vi "Main_FPGA 5.vi"() -> ()   [LabVIEW 2015]
uses:
  <vilib>/rvi/Emulation/niFpgaGetClockAttributes.vi
  <vilib>/rvi/Emulation/niFpgaSctlEmulationGetInTimedLoop.vi
  <vilib>/rvi/Emulation/niFpgaEmulationReportErrorSimple.vi
  <vilib>/rvi/Emulation/niFpgaProcessEmulError.vi
  <vilib>/rvi/eio/common/nirviEmuTemplateMethod_errors.vi
  <vilib>/rvi/interface/RandomDataEmulation/niFpgaRandomDataHandleErrors.vi
  <vilib>/rvi/Emulation/niFpgaCriticalErrorInLSC.vi
  <vilib>/eio/EIONode/EIONode.xnode
  <vilib>/rvi/DataTransferAndStorage/Container/XNode/niFpgaContainer.xnode
  <vilib>/rvi/interface/RandomDataEmulation/nirviRandomDataFpgaReadWriteTemplate.vi
panel:
  out "Loop delay (us)":u32
  out "Chassis Temperature":sgl
  out "FPGA Error":errorcluster
  out "Finished":bool
  in  "Stop":bool
  out "Module Underflow":bool
  out "DMA FIFO Full":bool
  out "Chan Count":bool
  out "Acq Loop Ticks":u32
  out "First Read":bool
  in  "Total Avail Channels":i32=4
  in  "Data Rate [S/s]":u32=1280
  in  "Acquisition Type":enum16{"Finite Samples", "Continuous Samples"}(ring)
  in  "Samps per Chan [Finite]":i32=5120
  in  "Number of Modules":i16=1
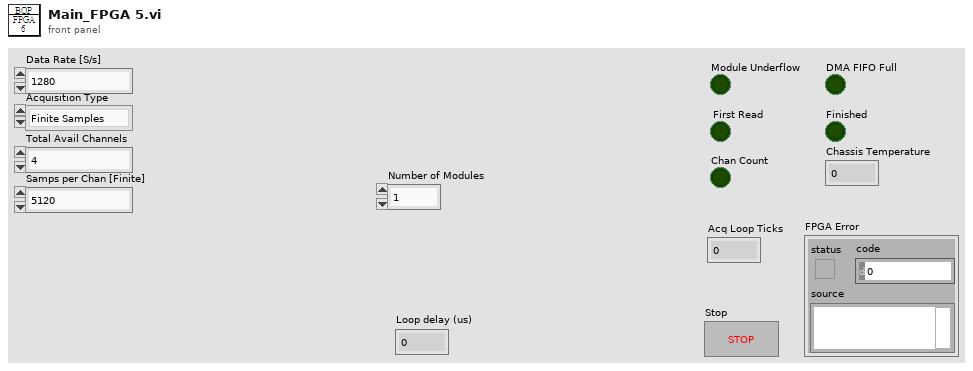
[diagram p1: front panel]
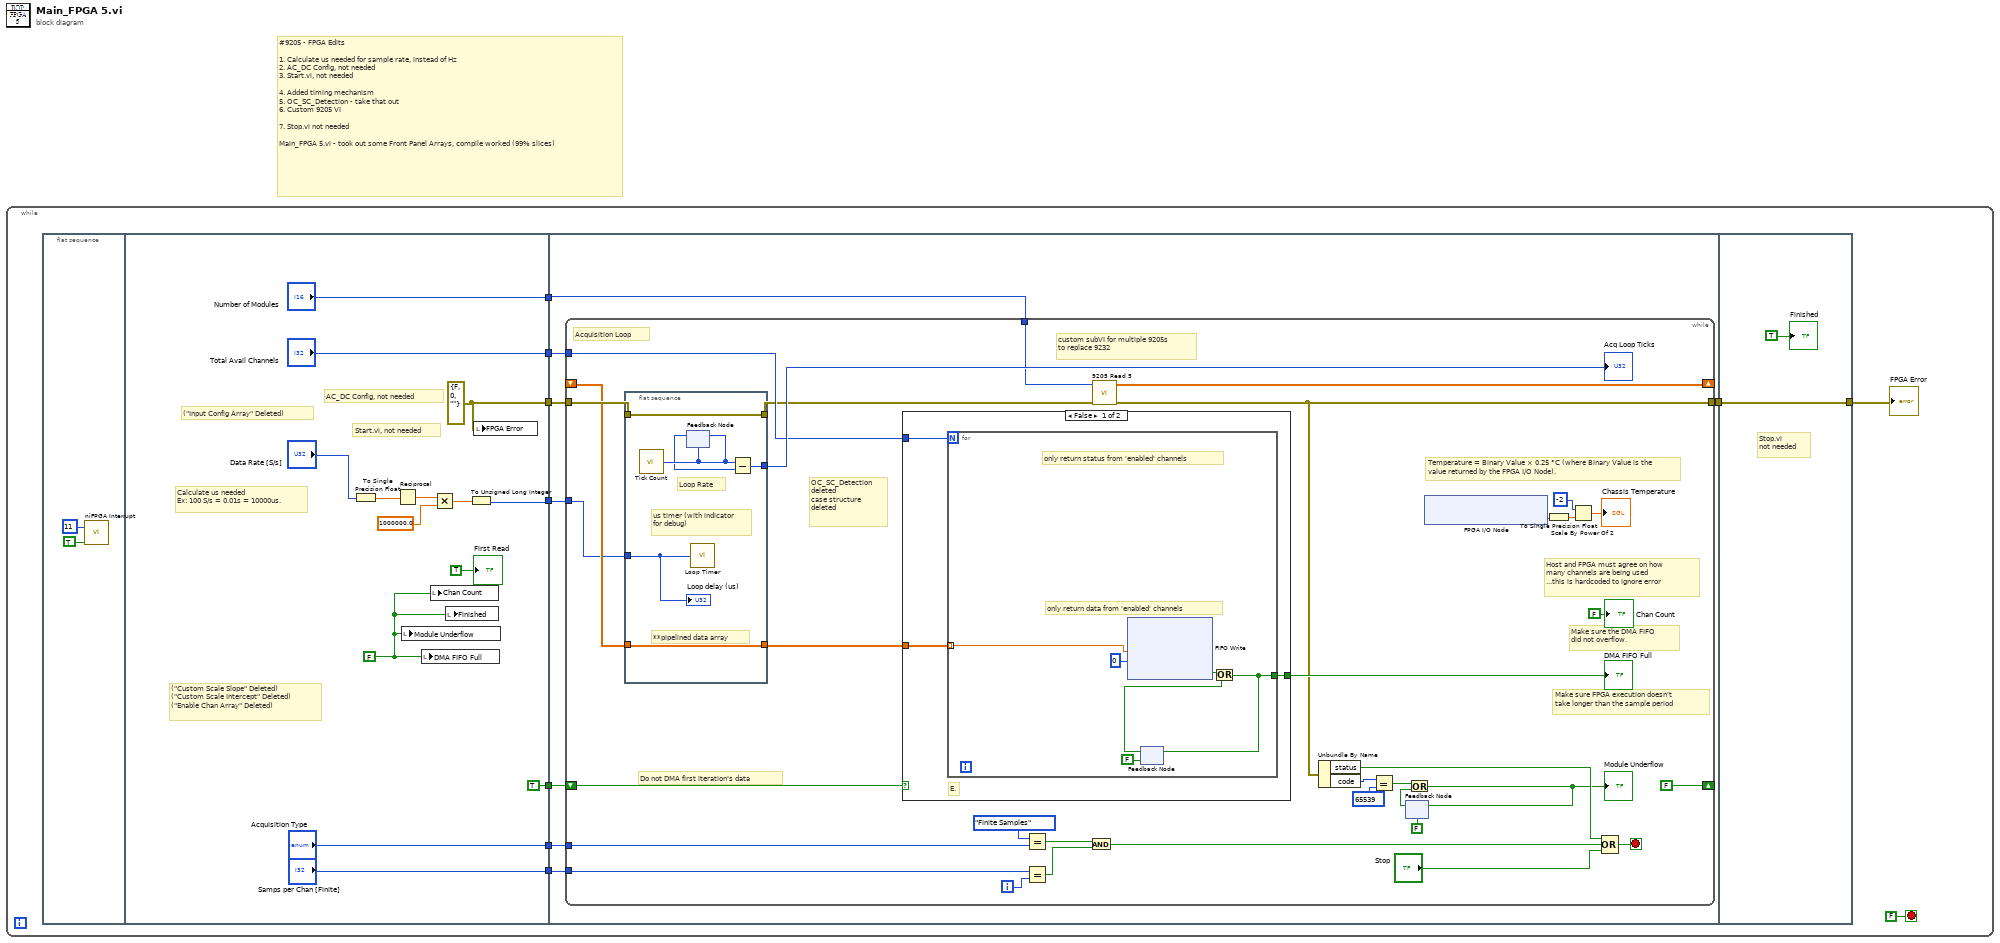
[diagram p0: block diagram]
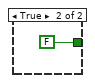
[diagram p2: hidden frame]
diagram:
  # "#9205 - FPGA Edits\n\n1. Calculate us needed for sample rate, instead of Hz\n2. AC_DC Config, not needed\n3. Start.vi, not needed\n\n4. Added timing mechanism\n5. OC_SC_Detection - take that out\n6. Custom 9205 VI\n\n7. Stop.vi not needed\n\nMain_FPGA 5.vi - took out some Front Panel Arrays, compile worked (99% slices)"
  n1 = while {
    stop <- FALSE stop-if-true
    n2 = flat-sequence {
      tunnel: [w19] -> w9
      tunnel: ["Acquisition Type"] -> w8
      tunnel: ["Samps per Chan [Finite]"] -> w7
      tunnel: ["Total Avail Channels"] -> w6
      tunnel: [TRUE ("t")] -> w5
      tunnel: ["Number of Modules"] -> w3
      tunnel: [w13] -> w1
      tunnel: w9 -> [w33]
      tunnel: w8 -> [w31]
      tunnel: w7 -> [w30]
      tunnel: w6 -> [w34]
      tunnel: w5 -> [w32]
      tunnel: [w29] -> w4
      tunnel: w3 -> [w28]
      tunnel: w1 -> [w27]
      tunnel: w4 -> [w85]
      tunnel: [w85] -> w2
      frame #0 {
        n3 = call <vilib>:"niFPGA Interrupt.vi"("Wait Until Cleared (F)"=TRUE ("Wait Until Cleared"), "IRQ Number (0)"=u8 11 ("IRQ Number")) -> ()  [unwired: 1 in]
      }
      frame #1 {
        w19 = errorcluster {"status"=FALSE, "code"=0, "source"=""} ("FPGA Error")
        w21 = FALSE ("Module Underflow")
        # "(\"Custom Scale Slope\" Deleted)\n(\"Custom Scale Intercept\" Deleted)\n(\"Enable Chan Array\" Deleted)"
        # "(\"Input Config Array\" Deleted)"
        # "Start.vi, not needed"
        # "AC_DC Config, not needed"
        # "Calculate us needed\nEx: 100 S/s = 0.01s = 10000us."
        n4 = To Single Precision Float(number="Data Rate [S/s]") -> (single precision float=w16:sgl)
        n5 = Reciprocal(x=w16) -> (1/x=w18:sgl)
        n6 = local write "Module Underflow"(w21) -> ()
        n7 = local write "DMA FIFO Full"(w21) -> ()
        n8 = local write "Chan Count"(w21) -> ()
        n9 = Multiply(x=w18, y=sgl 1000000.0) -> (x*y=w14:sgl)
        n10 = local write "Finished"(w21) -> ()
        n11 = To Unsigned Long Integer(number=w14) -> (unsigned 32bit integer=w13:u32)
        n12 = local write "FPGA Error"(w19) -> ()
        "First Read" <- TRUE ("First Read")
      }
      frame #2 {
        n13 = while {
          tunnel: w33 -> [w62]
          tunnel: [w37] -> w29
          tunnel: w31 -> [w64]
          tunnel: w30 -> [w63]
          shift-right: [w35] -> _
          shift-left: _ -> [w60]
          tunnel: w34 -> [w44]
          shift-right: [FALSE ("t")] -> _
          shift-left: w32 -> [w47]
          tunnel: w28 -> [w36]
          tunnel: w27 -> [w39]
          i -> [w58]
          stop <- w67 stop-if-true
          # "custom subVI for multiple 9205s\nto replace 9232"
          # "OC_SC_Detection\ndeleted\ncase structure\ndeleted"
          # "Temperature = Binary Value × 0.25 °C (where Binary Value is the value returned by the FPGA I/O Node)."
          # "Do not DMA first iteration's data"
          # "Acquisition Loop"
          # "Host and FPGA must agree on how \nmany channels are being used\n...this is hardcoded to ignore error"
          # "Make sure the DMA FIFO\ndid not overflow."
          # "Make sure FPGA execution doesn't\ntake longer than the sample period"
          n14 = flat-sequence {
            tunnel: [w84] -> w38
            tunnel: w62 -> [w84]
            tunnel: [w81] -> w61
            tunnel: w60 -> [w80]
            tunnel: [w80] -> w45
            tunnel: w39 -> [w79]
            frame #0 {
              # "us timer (with indicator\nfor debug)"
              # "**pipelined data array"
              # "Loop Rate"
              n15 = call "Tick Count"() -> ("Tick Count(Ticks)"=w83:u32)
              n16 = feedback-in #1(w83) -> ()
              n17 = feedback #1(w83) -> (w82:u32)
              n18 = call "Loop Timer"("Count(uSec)"=w79) -> ()  [unwired: 1 out]
              n19 = Subtract(x=w83, y=w82) -> (x-y=w81:u32)
              "Loop delay (us)" <- w79
            }
          }
          n20 = case shown="False" w47 {
            tunnel: [w71 FALSE] -> w46
            tunnel: w45 -> [w70 _]
            tunnel: w44 -> [w69 _]
            frame False {
              # "E."
              n21 = for {
                N: w69 -> [_]
                tunnel: [w76] -> w71
                tunnel: w70 -> [w75] mode=indexing
                # "only return status from 'enabled' channels"
                # "only return data from 'enabled' channels"
                n22 = xnode ("FIFO Write")("Element"=w75, "Timeout"=0) -> ("Timed Out?"=w72:bool)  [unwired: 1 in, 1 out]
                n23 = feedback #2(FALSE) -> (w77:bool)
                n24 = Or(x=w72, y=w77) -> (x .or. y?=w76:bool)
                n25 = feedback-in #2(w76) -> ()
              }
            }
            frame True {
            }
          }
          "DMA FIFO Full" <- w46
          n26 = Equal?(x=enum16{"Finite Samples", "Continuous Samples"}."Finite Samples" ("y"), y=w64) -> (x = y?=w52:bool)
          n27 = Equal?(x=w63, y=w58) -> (x = y?=w51:bool)
          n28 = And(x=w52, y=w51) -> (x .and. y?=w50:bool)
          n29 = call "9205 Read 5.vi"("error in"=w38, "Module Config Selector"=w36) -> ("error out"=w37:errorcluster, "Data Array"=w35:sgl[])  [unwired: 8 in]
          n30 = Unbundle By Name(w37) -> ("status"=w57:bool, "code"=w65:i32)
          n31 = Equal?(x=w65, y=65539) -> (x = y?=w54:bool)
          n32 = feedback #3(FALSE) -> (w56:bool)
          n33 = Or(x=w54, y=w56) -> (x .or. y?=w53:bool)
          "Module Underflow" <- w53
          n34 = feedback-in #3(w53) -> ()
          n35 = xnode "FPGA I/O Node"() -> ("Chassis Temperature"=w41:i16)  [unwired: 1 in, 1 out]
          n36 = To Single Precision Float(number=w41) -> (single precision float=w43:sgl)
          n37 = Scale By Power Of 2(n=i16 -2, x=w43) -> (x*2^n=→"Chassis Temperature":sgl)
          n38 = Compound Arithmetic op=OR(w57, w50, "Stop") -> (w67:bool)
          "Chan Count" <- FALSE ("Chan Count")
          "Acq Loop Ticks" <- w61
        }
      }
      frame #3 {
        # "Stop.vi\nnot needed"
        "Finished" <- TRUE ("Finished")
      }
    }
    "FPGA Error" <- w2
  }
